vi "Set Port.vi"(10 "Port":u16, 11 "Request in":refnum<class "Request.lvclass">) -> (3 "Request out":refnum<class "Request.lvclass">)   [LabVIEW 2020, in "OAuth2.lvlib" / "Request.lvclass"]
uses:
  Request.lvclass
  Request.lvclass/Request.ctl
  <vilib>/IlluminatedG/lv-stream/URI/URI.lvclass
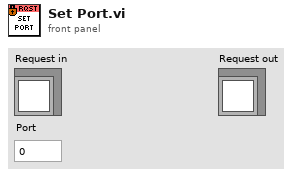
[diagram p1: front panel]
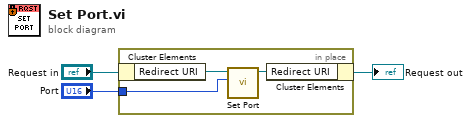
[diagram p0: block diagram]
diagram:
  n1 = in-place {
    in-place-border: "Port" -> [w4]
    n2 = in-place-cluster #1("Request in") -> ("Redirect URI"=w6:refnum<class "URI.lvclass">)
    n3 = call <vilib>:"Set Port.vi"("Port"=w4, "URI in"=w6) -> ("URI out"=w5:refnum<class "URI.lvclass">)  [unwired: 8 in, 1 out]
    n4 = in-place-cluster #1("Redirect URI"=w5) -> (→"Request out":refnum<class "Request.lvclass">)
  }
